vi "坐标偏移补偿.vi"(0 "布线前甩线":string[][](table), 5 "布线后甩线":string[][](table), 7 "布线点位":string[][](table)) -> (4 "布线前甩线矫正后":string[][](table), 6 "布线后甩线矫正后":string[][](table), 8 "布线点矫正后":string[][](table))   [LabVIEW 2014]
uses:
  Controls/XYPos.ctl
  Global.vi
panel:
  out "布线后偏移":T1[][](array[typedef]) {"X" format="%#.3f"}
  out "布线点偏移":cluster{"Pos":T1, "Pos":T1}[][](array[cluster]) {"Pos"."X" format="%#.3f"; "Pos"."X" format="%#.3f"}
  out "布线前偏移":T1[][](array[typedef]) {"X" format="%#.3f"}
  out "布线点":cluster{"Pos":T1, "Pos":T1}[][](array[cluster]) {"Pos"."X" format="%#.3f"; "Pos"."X" format="%#.3f"}
  out "布线后点":T1[][](array[typedef]) {"X" format="%#.3f"}
  out "布线前点":T1[][](array[typedef]) {"X" format="%#.3f"}
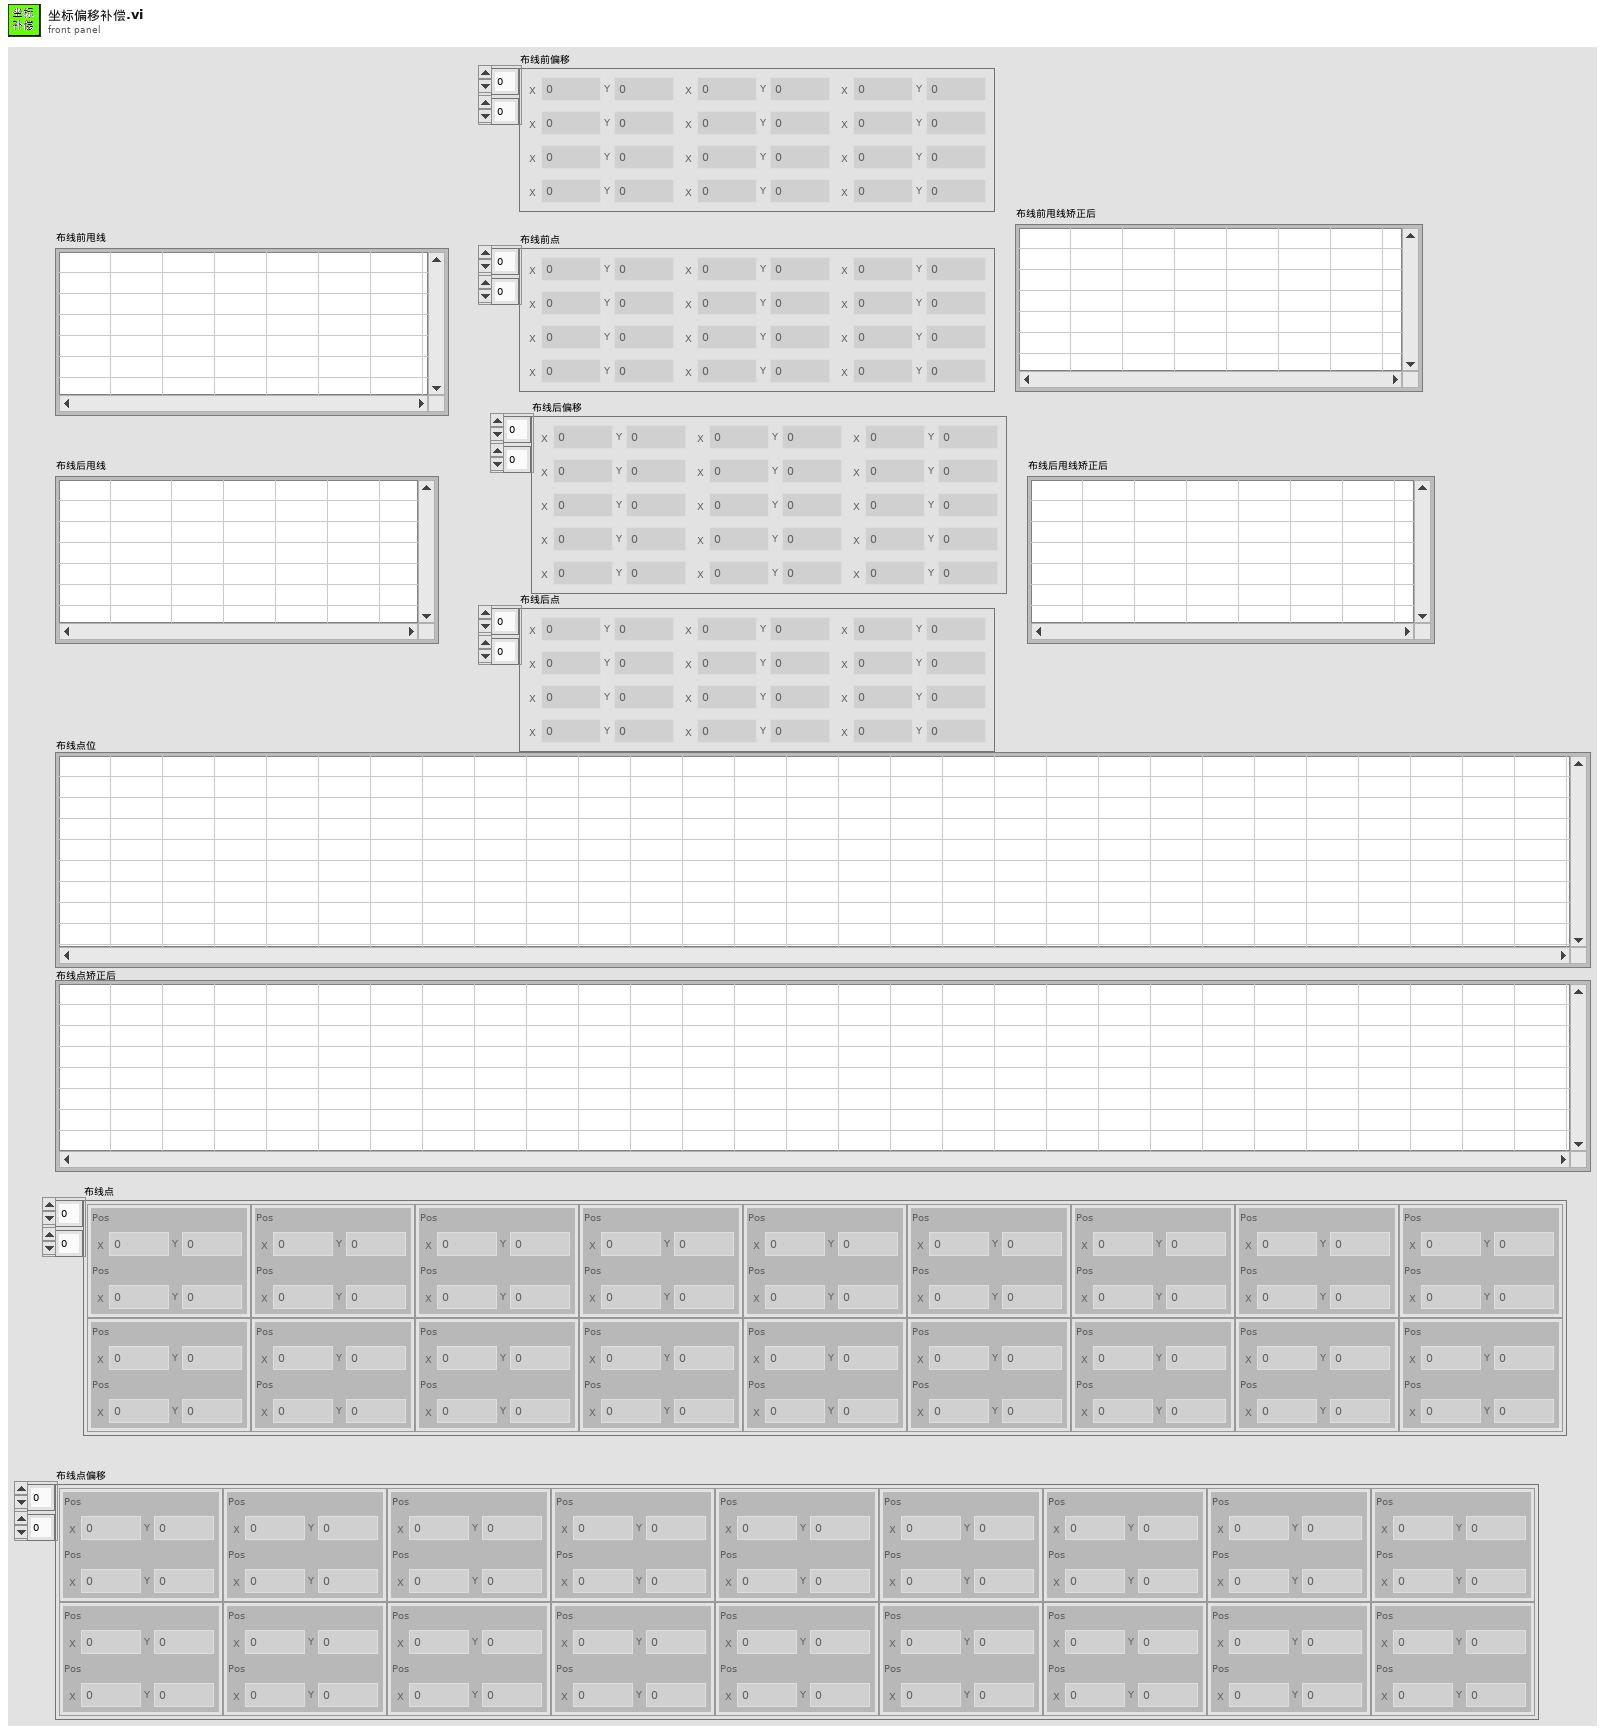
[diagram p1: front panel]
types:
  T1 = typedef "XYPos.ctl" = cluster{"X":dbl, "Y":dbl}
  T2 = cluster{"mark 1 ":cluster{"X":dbl, "Y":dbl}, "mark 2":cluster{"X":dbl, "Y":dbl}}
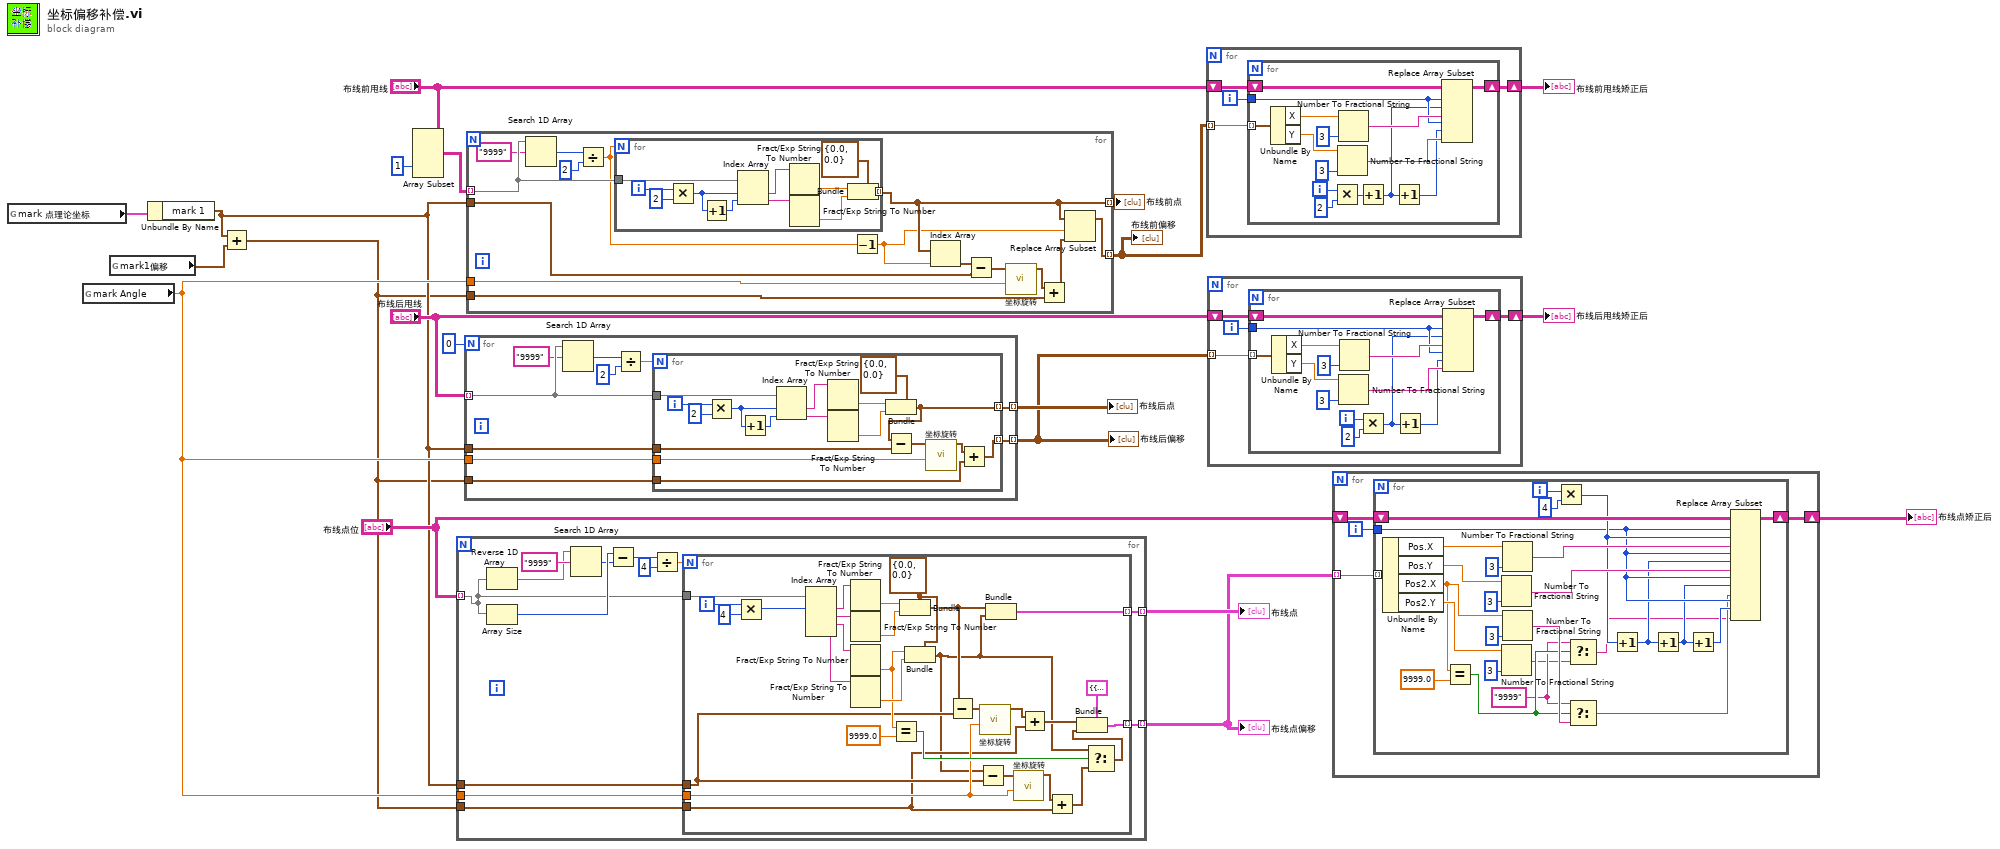
[diagram p0: block diagram]
diagram:
  n1 = global read "Global.vi" "mark 点理论坐标"() -> (w7:T2)
  n2 = global read "Global.vi" "mark Angle"() -> (w11:dbl)
  n3 = global read "Global.vi" "mark1偏移"() -> (w6:T1)
  n4 = Unbundle By Name(w7) -> ("mark 1"=w5:cluster{"X":dbl, "Y":dbl})
  n5 = Add(x=w5, y=w6) -> (x+y=w4:T1)
  n6 = Array Subset(array="布线前甩线", index (col)=1 ("索引")) -> (w8:string[][])  [unwired: 3 in]
  n7 = for {
    tunnel: "布线点位" -> [w24] mode=indexing
    tunnel: [w26] -> w14 mode=indexing
    tunnel: [w25] -> w13 mode=indexing
    tunnel: w11 -> [w23]
    tunnel: w5 -> [w22]
    tunnel: w4 -> [w21]
    n8 = Reverse 1D Array(array=w24) -> (reversed array=w30:string[])
    n9 = Array Size(array=w24) -> (size(s)=w29:i32)
    n10 = Search 1D Array(1D array=w30, element="9999" ("元素")) -> (index of element=w28:i32)  [unwired: 1 in]
    n11 = Subtract(x=w29, y=w28) -> (x-y=w27:i32)
    n12 = Divide(x=w27, y=4) -> (x/y=w32:dbl)
    n13 = for {
      N: w32 -> [_]
      tunnel: w24 -> [w63]
      tunnel: [w51] -> w26 mode=indexing
      tunnel: [w50] -> w25 mode=indexing
      tunnel: w23 -> [w39]
      tunnel: w22 -> [w38]
      tunnel: w21 -> [w36]
      i -> [w62]
      w52 = T1 {"X"=0.0, "Y"=0.0} ("Pos")
      n14 = Multiply(x=w62, y=4) -> (x*y=w60:i32)
      n15 = Index Array(array=w63, index #1=w60) -> (element #1=w59:string, element #2=w58:string, element #3=w54:string, element #4=w53:string)  [unwired: 3 in]
      n16 = Fract/Exp String To Number(string=w59) -> (number=w57:dbl)  [unwired: 3 in, 1 out]
      n17 = Fract/Exp String To Number(string=w58) -> (number=w56:dbl)  [unwired: 3 in, 1 out]
      n18 = Fract/Exp String To Number(string=w54) -> (number=w49:dbl)  [unwired: 3 in, 1 out]
      n19 = Fract/Exp String To Number(string=w53) -> (number=w55:dbl)  [unwired: 3 in, 1 out]
      n20 = Equal?(x=w49, y=9999.0) -> (x = y?=w47:bool)
      n21 = Bundle(cluster=w52, "X"=w57, "Y"=w56) -> (w35:T1)
      n22 = Bundle(cluster=w52, "X"=w49, "Y"=w55) -> (w34:T1)
      n23 = Subtract(x=w35, y=w38) -> (x-y=w43:T1)
      n24 = Subtract(x=w34, y=w38) -> (x-y=w41:T1)
      n25 = call "坐标旋转.vi"("旋转角度(单位°)"=w39, "dtx,dty In"=w43) -> ("dtx,dty Out"=w44:cluster{"X":dbl, "Y":dbl})  [unwired: 9 in]
      n26 = Bundle("Pos"=w35, "Pos"=w34) -> (w51:cluster{"Pos":T1, "Pos":T1})  [unwired: 1 in]
      n27 = call "坐标旋转.vi"("旋转角度(单位°)"=w39, "dtx,dty In"=w41) -> ("dtx,dty Out"=w40:cluster{"X":dbl, "Y":dbl})  [unwired: 9 in]
      n28 = Add(x=w44, y=w36) -> (x+y=w42:T1)
      n29 = Add(x=w40, y=w36) -> (x+y=w37:T1)
      n30 = Select(t=w34, s=w47, f=w37) -> (s? t:f=w46:T1)
      n31 = Bundle(cluster=cluster{"Pos":T1, "Pos2":T1} {"Pos"={"X"=0.0, "Y"=0.0}, "Pos2"={"X"=0.0, "Y"=0.0}}, "Pos"=w42, "Pos2"=w46) -> (w50:cluster{"Pos":T1, "Pos2":T1})
    }
  }
  "布线点" <- w14
  "布线点偏移" <- w13
  n32 = for {
    N: 0 -> [_]
    tunnel: "布线后甩线" -> [w70] mode=indexing
    tunnel: [w71] -> w17 mode=indexing
    tunnel: w11 -> [w67]
    tunnel: w5 -> [w66]
    tunnel: w4 -> [w65]
    tunnel: [w64] -> w3 mode=indexing
    n33 = Search 1D Array(1D array=w70, element="9999" ("元素")) -> (index of element=w68:i32)  [unwired: 1 in]
    n34 = Divide(x=w68, y=2) -> (x/y=w72:dbl)
    n35 = for {
      N: w72 -> [_]
      tunnel: w70 -> [w90]
      tunnel: [w78] -> w71 mode=indexing
      tunnel: w67 -> [w75]
      tunnel: w66 -> [w77]
      tunnel: w65 -> [w76]
      tunnel: [w74] -> w64 mode=indexing
      i -> [w89]
      n36 = Multiply(x=w89, y=2) -> (x*y=w86:i32)
      n37 = Increment(x=w86) -> (x+1=w87:i32)
      n38 = Index Array(array=w90, index #1=w86, index #2=w87) -> (element #1=w85:string, element #2=w84:string)
      n39 = Fract/Exp String To Number(string=w85) -> (number=w83:dbl)  [unwired: 3 in, 1 out]
      n40 = Fract/Exp String To Number(string=w84) -> (number=w82:dbl)  [unwired: 3 in, 1 out]
      n41 = Bundle(cluster=T1 {"X"=0.0, "Y"=0.0} ("Pos"), "X"=w83, "Y"=w82) -> (w78:T1)
      n42 = Subtract(x=w78, y=w77) -> (x-y=w79:T1)
      n43 = call "坐标旋转.vi"("旋转角度(单位°)"=w75, "dtx,dty In"=w79) -> ("dtx,dty Out"=w80:cluster{"X":dbl, "Y":dbl})  [unwired: 9 in]
      n44 = Add(x=w80, y=w76) -> (x+y=w74:T1)
    }
  }
  "布线后点" <- w17
  "布线后偏移" <- w3
  n45 = for {
    tunnel: w8 -> [w104] mode=indexing
    tunnel: [w95] -> w20 mode=indexing
    tunnel: [w98] -> w1 mode=indexing
    tunnel: w11 -> [w101]
    tunnel: w5 -> [w100]
    tunnel: w4 -> [w99]
    n46 = Search 1D Array(1D array=w104, element="9999" ("元素")) -> (index of element=w102:i32)  [unwired: 1 in]
    n47 = Divide(x=w102, y=2) -> (x/y=w94:dbl)
    n48 = for {
      N: w94 -> [_]
      tunnel: w104 -> [w116]
      tunnel: [w106] -> w95 mode=indexing
      i -> [w115]
      n49 = Multiply(x=w115, y=2) -> (x*y=w112:i32)
      n50 = Increment(x=w112) -> (x+1=w113:i32)
      n51 = Index Array(array=w116, index #1=w112, index #2=w113) -> (element #1=w111:string, element #2=w110:string)
      n52 = Fract/Exp String To Number(string=w111) -> (number=w109:dbl)  [unwired: 3 in, 1 out]
      n53 = Fract/Exp String To Number(string=w110) -> (number=w108:dbl)  [unwired: 3 in, 1 out]
      n54 = Bundle(cluster=T1 {"X"=0.0, "Y"=0.0} ("Pos"), "X"=w109, "Y"=w108) -> (w106:T1)
    }
    n55 = Decrement(x=w94) -> (x-1=w91:dbl)
    n56 = Index Array(array=w95, index=w91) -> (element=w93:T1)
    n57 = Subtract(x=w93, y=w100) -> (x-y=w97:T1)
    n58 = call "坐标旋转.vi"("旋转角度(单位°)"=w101, "dtx,dty In"=w97) -> ("dtx,dty Out"=w96:cluster{"X":dbl, "Y":dbl})  [unwired: 9 in]
    n59 = Add(x=w96, y=w99) -> (x+y=w92:T1)
    n60 = Replace Array Subset(array=w95, new element=w92, index=w91) -> (w98:T1[])
  }
  "布线前点" <- w20
  "布线前偏移" <- w1
  n61 = for {
    shift-right: [w118] -> w19
    shift-left: "布线前甩线" -> [w119]
    tunnel: w1 -> [w117] mode=indexing
    i -> [w120]
    n62 = for {
      tunnel: w120 -> [w128]
      shift-right: [w130] -> w118
      shift-left: w119 -> [w131]
      tunnel: w117 -> [w123] mode=indexing
      i -> [w126]
      n63 = Unbundle By Name(w123) -> ("X"=w135:dbl, "Y"=w132:dbl)
      n64 = Multiply(x=w126, y=2) -> (x*y=w122:i32)
      n65 = Number To Fractional String(number=w132, precision (6)=i16 3 ("精度(6)")) -> (F-format string=w127:string)  [unwired: 2 in]
      n66 = Number To Fractional String(number=w135, precision (6)=i16 3 ("精度(6)")) -> (F-format string=w129:string)  [unwired: 2 in]
      n67 = Increment(x=w122) -> (x+1=w121:i32)
      n68 = Increment(x=w121) -> (x+1=w124:i32)
      n69 = Replace Array Subset(array=w131, new element #1=w129, index (row) #1=w128, index (col) #1=w121, new element #2=w127, index (row) #2=w128, index (col) #2=w124) -> (w130:string[][])
    }
  }
  "布线前甩线矫正后" <- w19
  n70 = for {
    shift-right: [w137] -> w15
    shift-left: "布线后甩线" -> [w138]
    tunnel: w3 -> [w136] mode=indexing
    i -> [w139]
    n71 = for {
      tunnel: w139 -> [w146]
      shift-right: [w148] -> w137
      shift-left: w138 -> [w149]
      tunnel: w136 -> [w140] mode=indexing
      i -> [w144]
      n72 = Unbundle By Name(w140) -> ("X"=w153:dbl, "Y"=w150:dbl)
      n73 = Number To Fractional String(number=w150, precision (6)=i16 3 ("精度(6)")) -> (F-format string=w145:string)  [unwired: 2 in]
      n74 = Number To Fractional String(number=w153, precision (6)=i16 3 ("精度(6)")) -> (F-format string=w147:string)  [unwired: 2 in]
      n75 = Multiply(x=w144, y=2) -> (x*y=w142:i32)
      n76 = Increment(x=w142) -> (x+1=w141:i32)
      n77 = Replace Array Subset(array=w149, new element #1=w147, index (row) #1=w146, index (col) #1=w142, new element #2=w145, index (row) #2=w146, index (col) #2=w141) -> (w148:string[][])
    }
  }
  "布线后甩线矫正后" <- w15
  n78 = for {
    tunnel: w13 -> [w156] mode=indexing
    shift-right: [w154] -> w12
    shift-left: "布线点位" -> [w155]
    i -> [w157]
    n79 = for {
      tunnel: w157 -> [w172]
      tunnel: w156 -> [w184] mode=indexing
      shift-right: [w178] -> w154
      shift-left: w155 -> [w179]
      i -> [w175]
      w160 = "9999"
      n80 = Unbundle By Name(w184) -> ("Pos.X"=w183:dbl, "Pos.Y"=w180:dbl, "Pos2.X"=w164:dbl, "Pos2.Y"=w166:dbl)
      n81 = Equal?(x=w164, y=9999.0) -> (x = y?=w161:bool)
      n82 = Number To Fractional String(number=w180, precision (6)=i16 3 ("精度(6)")) -> (F-format string=w176:string)  [unwired: 2 in]
      n83 = Number To Fractional String(number=w166, precision (6)=i16 3 ("精度(6)")) -> (F-format string=w159:string)  [unwired: 2 in]
      n84 = Number To Fractional String(number=w183, precision (6)=i16 3 ("精度(6)")) -> (F-format string=w177:string)  [unwired: 2 in]
      n85 = Number To Fractional String(number=w164, precision (6)=i16 3 ("精度(6)")) -> (F-format string=w163:string)  [unwired: 2 in]
      n86 = Multiply(x=w175, y=4) -> (x*y=w173:i32)
      n87 = Select(t=w160, s=w161, f=w159) -> (s? t:f=w158:string)
      n88 = Select(t=w160, s=w161, f=w163) -> (s? t:f=w162:string)
      n89 = Increment(x=w173) -> (x+1=w169:i32)
      n90 = Increment(x=w169) -> (x+1=w168:i32)
      n91 = Increment(x=w168) -> (x+1=w167:i32)
      n92 = Replace Array Subset(array=w179, new element #1=w177, index (row) #1=w172, index (col) #1=w173, new element #2=w176, index (row) #2=w172, index (col) #2=w169, new element #3=w162, index (row) #3=w172, index (col) #3=w168, new element #4=w158, index (row) #4=w172, index (col) #4=w167) -> (w178:string[][])
    }
  }
  "布线点矫正后" <- w12
